vi "Main.vi"() -> ()   [LabVIEW 2022 SP3]
doc: "Use this template to build a simple state machine design pattern. Each state executes code and determines which state to transition to."
uses:
  controls/State.ctl
  controls/Data.ctl
  Acuisition.lvlib
  controls/TaskState.ctl
panel:
  in  "PID Controller":bool
  in  "Logging":bool
  in  "Acquisition":bool
  in  "Exit":bool
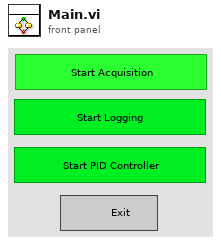
[diagram p1: front panel]
types:
  T1 = typedef "TaskState.ctl" = enum16{"Ready", "Running", "Stopped"}
  T2 = typedef "Data.ctl" = cluster{"Boolean <Replace Me>":bool, "String <Replace Me>":string, "Numeric <Replace Me>":dbl}
  T3 = typedef "State.ctl" = enum16{"Initialize", "Wait for Event", "Acquire", "Log", "Control", "Exit"}
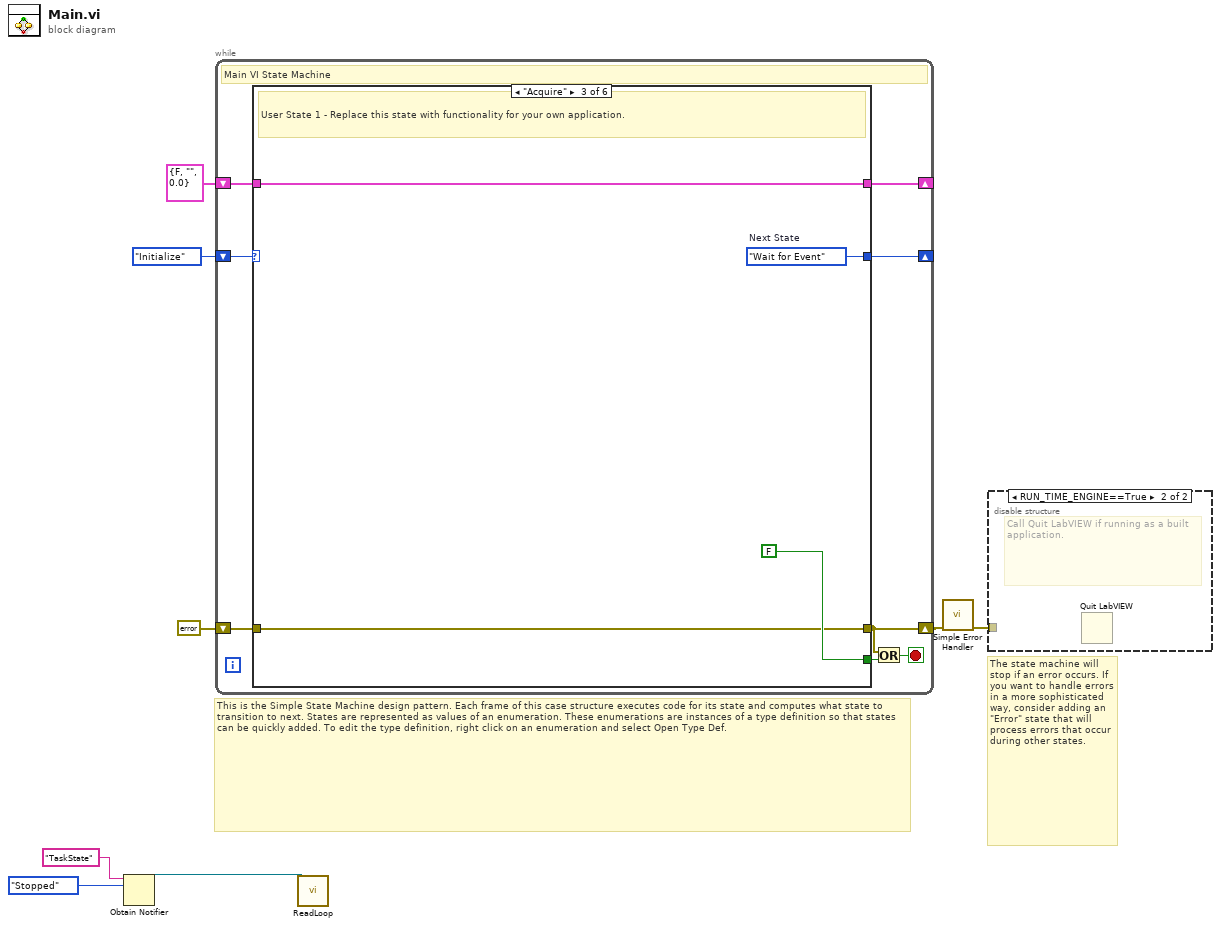
[diagram p0: block diagram]
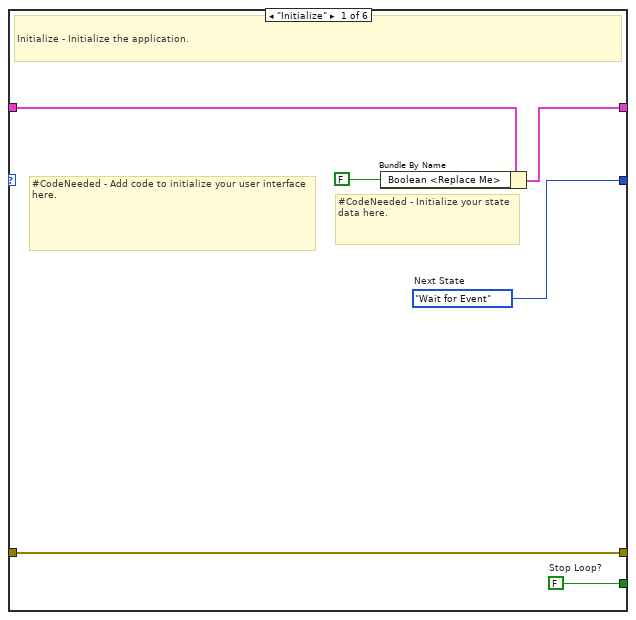
[diagram p3: hidden frame]
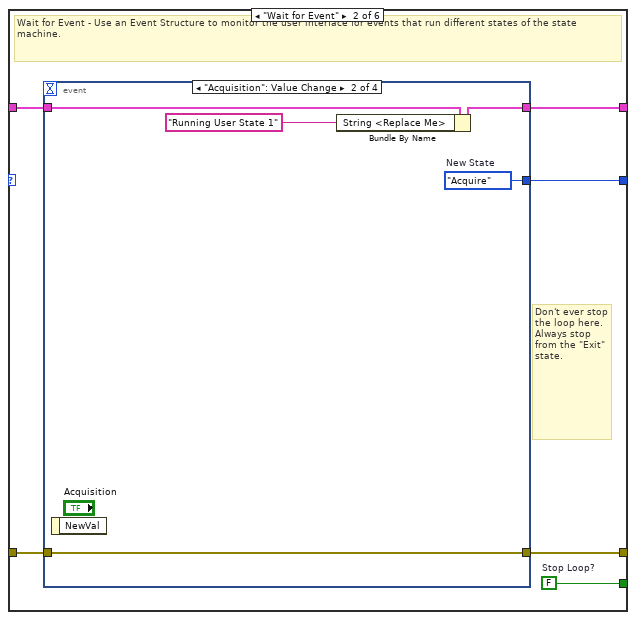
[diagram p4: hidden frame]
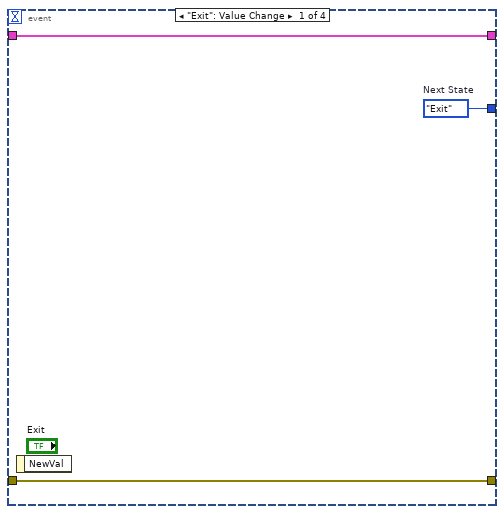
[diagram p5: hidden frame]
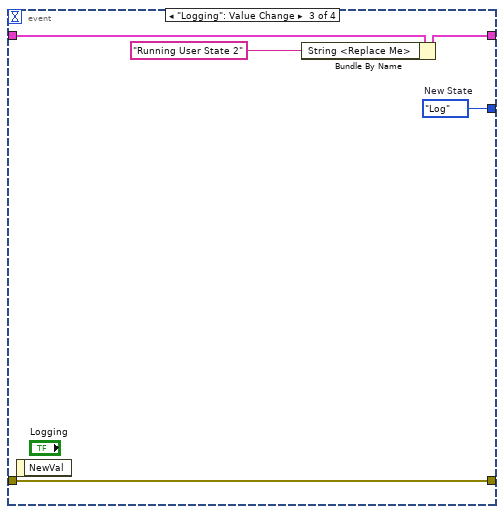
[diagram p6: hidden frame]
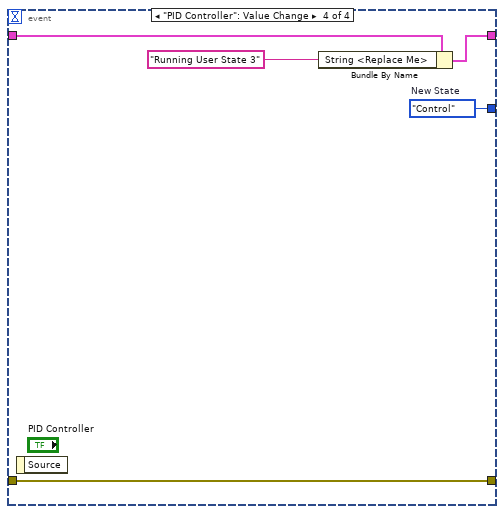
[diagram p7: hidden frame]
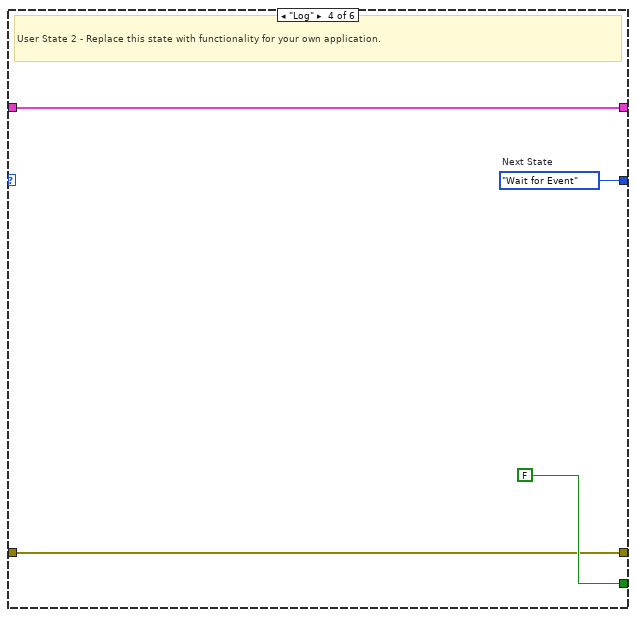
[diagram p8: hidden frame]
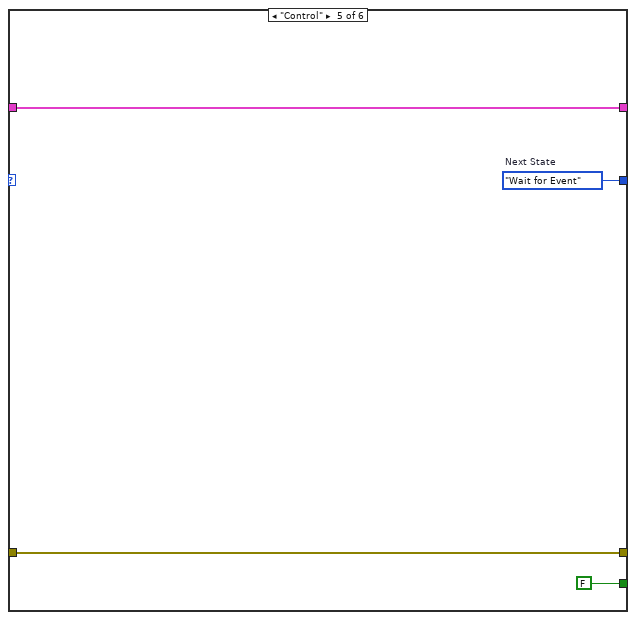
[diagram p9: hidden frame]
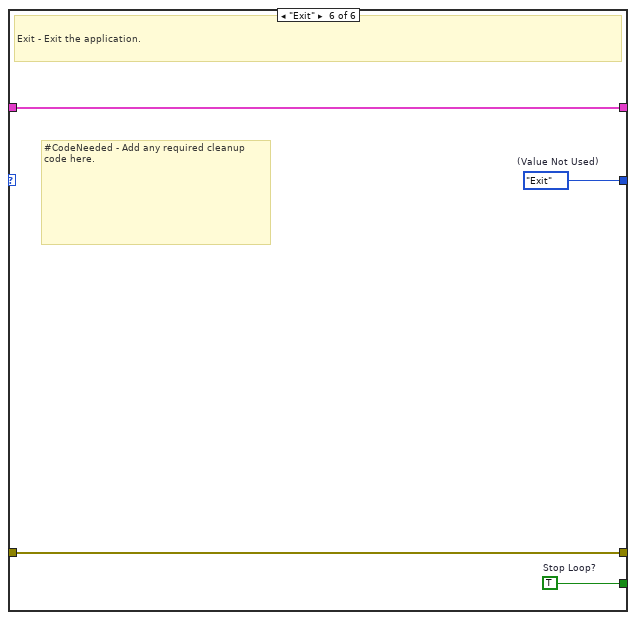
[diagram p10: hidden frame]
diagram:
  # "The state machine will stop if an error occurs. If you want to handle errors in a more sophisticated way, consider adding an \"Error\" state that will process errors that occur during other states."
  # "This is the Simple State Machine design pattern. Each frame of this case structure executes code for its state and computes what state to transition to next. States are represented as values of an enumeration. These enumerations are instances of a type definition so that states can be quickly added. To edit the type definition, right click on an enumeration and select Open Type Def."
  n1 = Obtain Notifier(name (unnamed)="TaskState", notification data type=TaskState."Stopped" ("States")) -> (notifier out=w1:refnum<notifier>)  [unwired: 2 in, 2 out]
  n2 = while {
    shift-right: [w15] -> _
    shift-left: State."Initialize" ("Initial State") -> [w16]
    shift-right: [w13] -> _
    shift-left: T2 {"Boolean <Replace Me>"=FALSE, "String <Replace Me>"="", "Numeric <Replace Me>"=0.0} ("Data") -> [w14]
    shift-right: [w9] -> w5
    shift-left: errorcluster {"status"=FALSE, "code"=0, "source"=""} ("error constant") -> [w12]
    stop <- w10 stop-if-true
    # "Main VI State Machine"
    n3 = case shown="\"Acquire\"" w16 {
      tunnel: [w22 w28 w50 w54 w56 w62] -> w15
      tunnel: [w21 w27 FALSE ("Stop Loop?") FALSE ("Stop Loop?") FALSE ("Stop Loop?") w60] -> w11
      tunnel: w14 -> [w20 w26 w47 w52 w57 w61]
      tunnel: [w19 w25 w47 w52 w57 w61] -> w13
      tunnel: w12 -> [w17 w24 w48 w51 w58 w59]
      tunnel: [w17 w23 w48 w51 w58 w59] -> w9
      frame "Initialize" {
        w21 = FALSE  # Stop Loop?
        w22 = State."Wait for Event"  # Next State
        # "#CodeNeeded - Initialize your state data here."
        # "#CodeNeeded - Add code to initialize your user interface here."
        # "Initialize - Initialize the application."
        n4 = Bundle By Name(cluster=w20, "Boolean <Replace Me>"=FALSE ("Replace_Me_Boolean")) -> (w19:T2)
      }
      frame "Wait for Event" {
        w27 = FALSE  # Stop Loop?
        # "Don't ever stop the loop here. Always stop from the \"Exit\" state."
        # "Wait for Event - Use an Event Structure to monitor the user interface for events that run different states of the state machine."
        n5 = event shown="[1] \"Acquisition\": Value Change" {
          selector: _ -> [_ _ _ _]
          dyn-events: _ -> [_ _ _ _]
          timeout: _ -> [_ _ _ _]
          tunnel: [w31 w32 w37 w42] -> w28
          tunnel: w26 -> [w30 w36 w41 w44]
          tunnel: [w30 w35 w40 w43] -> w25
          tunnel: w24 -> [w29 w33 w38 w46]
          tunnel: [w29 w33 w38 w46] -> w23
          event "Exit": Value Change {
            w31 = State."Exit"  # Next State
            n6 = event-data() -> ()  [unwired: 1 in, 1 out]
          }
          event "Acquisition": Value Change {
            w32 = State."Acquire"  # New State
            n7 = event-data() -> ()  [unwired: 1 in, 1 out]
            n8 = Bundle By Name(cluster=w36, "String <Replace Me>"="Running User State 1" ("Running User State 1")) -> (w35:T2)
          }
          event "Logging": Value Change {
            w37 = State."Log"  # New State
            n9 = event-data() -> ()  [unwired: 1 in, 1 out]
            n10 = Bundle By Name(cluster=w41, "String <Replace Me>"="Running User State 2" ("Running User State 2")) -> (w40:T2)
          }
          event "PID Controller": Value Change {
            w42 = State."Control"  # New State
            n11 = event-data() -> ()  [unwired: 1 in, 1 out]
            n12 = Bundle By Name(cluster=w44, "String <Replace Me>"="Running User State 3" ("Running User State 2")) -> (w43:T2)
          }
        }
      }
      frame "Acquire" {
        w50 = State."Wait for Event"  # Next State
        # "User State 1 - Replace this state with functionality for your own application."
      }
      frame "Log" {
        w54 = State."Wait for Event"  # Next State
        # "User State 2 - Replace this state with functionality for your own application."
      }
      frame "Control" {
        w56 = State."Wait for Event"  # Next State
      }
      frame "Exit" {
        w60 = TRUE  # Stop Loop?
        w62 = State."Exit"  # (Value Not Used)
        # "#CodeNeeded - Add any required cleanup code here."
        # "Exit - Exit the application."
      }
    }
    n13 = Or(x=w9, y=w11) -> (x .or. y?=w10:bool)
  }
  n14 = call "ReadLoop.vi"("notifier"=w1) -> ()  [unwired: 11 in]
  n15 = call <vilib>:"Simple Error Handler.vi"("error in (no error)"=w5) -> ("error out"=w4:errorcluster)  [unwired: 4 in, 4 out]
  n16 = disable-structure shown="RUN_TIME_ENGINE==True" {
    disable-tunnel: w4 -> [_ _]
    frame condition #0 (active) {
    }
    frame condition #1 {
      # "Call Quit LabVIEW if running as a built application."
      n17 = Quit LabVIEW() -> ()  [unwired: 1 in]
    }
  }
